vi "SetPosHardware.vi"(6 "RealMove":dbl, 7 "SingleMove?":bool, 8 "error in (no error)":errorcluster, 9 "Axis 1":string, 10 "FirstMove":dbl, 11 "NewportXPS in":refnum<class "NewportXPS.lvclass">) -> (0 "error out":errorcluster, 3 "NewportXPS out":refnum<class "NewportXPS.lvclass">)   [LabVIEW 2020, in "NewportXPS.lvclass"]
uses:
  NewportXPS.lvclass
  NewportXPS.lvclass/NewportXPS.ctl
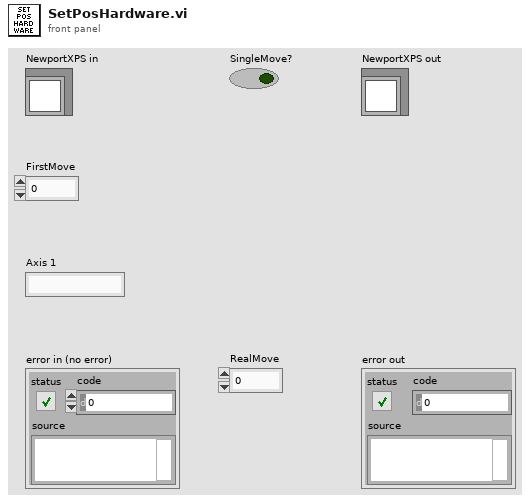
[diagram p1: front panel]
types:
  T1 = cluster{"connection TCP":refnum<k5>, "LogTo File":bool, "Log File refnum":refnum<file>, "no error if error log":bool}
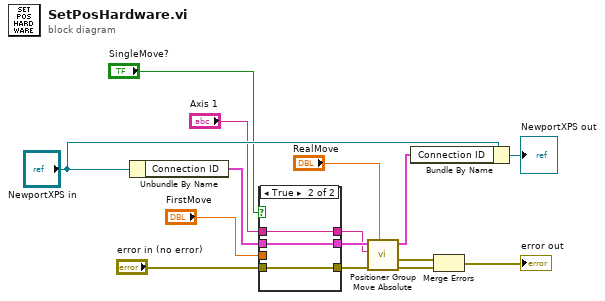
[diagram p0: block diagram]
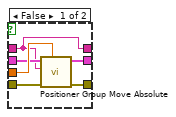
[diagram p2: hidden frame]
diagram:
  n1 = Unbundle By Name("NewportXPS in") -> ("Connection ID"=w14:T1)
  n2 = case shown="True" "SingleMove?" {
    tunnel: "Axis 1" -> [w16 w22]
    tunnel: "error in (no error)" -> [w21 w24]
    tunnel: [w20 w24] -> w12
    tunnel: [w19 w23] -> w13
    tunnel: "FirstMove" -> [w18 _]
    tunnel: w14 -> [w17 w23]
    tunnel: [w16 w22] -> w1
    frame False {
      n3 = call "Positioner Group Move Absolute.vi"("Target Position (units)"=w18, "error in (no error)"=w21, "Positioner Name (250 c max)"=w16, "connection ID in"=w17) -> ("error out"=w20:errorcluster, "connection ID out"=w19:T1)  [unwired: 5 in, 1 out]
    }
    frame True {
    }
  }
  n4 = call "Positioner Group Move Absolute.vi"("Target Position (units)"="RealMove", "error in (no error)"=w12, "Positioner Name (250 c max)"=w1, "connection ID in"=w13) -> ("error out"=w3:errorcluster, "XPS error out"=w2:errorcluster, "connection ID out"=w15:T1)  [unwired: 5 in]
  n5 = Bundle By Name(cluster="NewportXPS in", "Connection ID"=w15) -> (→"NewportXPS out":refnum<class "NewportXPS.lvclass">)
  n6 = Merge Errors(w2, w3) -> (→"error out":errorcluster)
